vi "DBC Get Msg Signal Quantity.vi"(10 "pMsgName":string, 11 "DBCHandle":u64) -> (2 "pMsgName out":string, 3 "function return":i32)   [LabVIEW 2010, in "dbc_parser.lvlib"]
doc: "int WINAPI DBC_GetMsgSignalQuantity(long long DBCHandle, char* pMsgName);"
uses:
  dbc_parser.lvlib
  USB2XXX/trunk/USB2XXX/USB2XXX/vs2019/Release/USB2XXX.dll
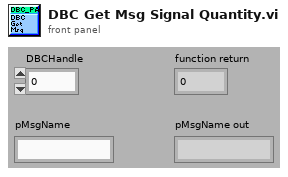
[diagram p1: front panel]
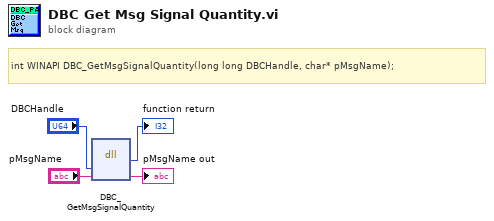
[diagram p0: block diagram]
diagram:
  # "int WINAPI DBC_GetMsgSignalQuantity(long long DBCHandle, char* pMsgName);"
  n1 = dll-call lib="E:/Projects/USB2XXX/trunk/USB2XXX/USB2XXX/vs2019/Release/USB2XXX.*" fn="DBC_GetMsgSignalQuantity"("DBCHandle"="DBCHandle", "pMsgName"="pMsgName") -> (→"function return":i32, "pMsgName"=→"pMsgName out":string)  [unwired: 4 in, 2 out]
